vi "niRFSTS Sequence Flow Obtain Session.vi"(0 "Session  Name ()":string, 1 "Include All Evaluations?":bool, 2 "Prepend Result Names?":bool, 5 "New Sequence File Path":path=path "C:/Users/QFE3320 VM/Desktop/CW1.seq", 7 "Template Path":path=path "C:/QFE3320/QFE3320_Template.seq", 9 "Limits File Path":path, 11 "error in (no error)":errorcluster, 12 "Use Existing Test Numbers?":bool) -> (4 "Session Handle":T1, 15 "error out":errorcluster)   [LabVIEW 2018, in "niRFSTS Sequence Flow.lvclass"]
doc: "This function initializes the measurement\n\nPass the function a name to obtain an active measurement handle"
uses:
  niRFSTS Sequence Flow.lvclass
  Typedefs/Session Handle.ctl
  C:/Sequence Automation/Plugins/Sequence Automation Session.lvlibp/Sequence Automation Session.lvclass
  niRFSTS Sequence Flow.lvclass/niRFSTS Sequence Flow.ctl
  Plugins/Sequence Automation Session.lvlibp/Sequence Automation Session.lvclass
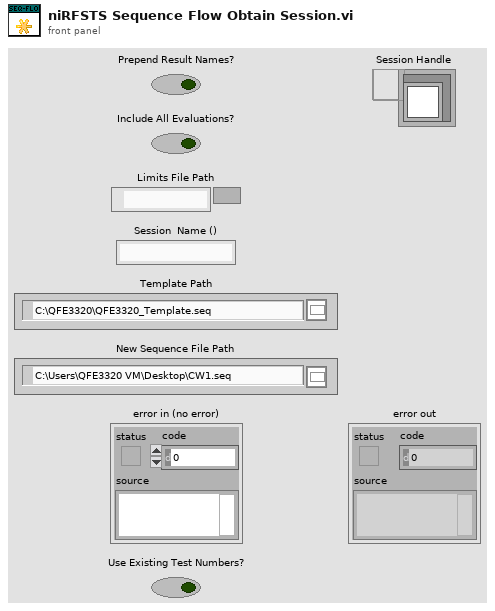
[diagram p1: front panel]
types:
  T1 = typedef "niRFSTS Sequence Flow.lvclass/Session Handle.ctl" = refnum<data-value>
  T2 = typedef "Sequence Automation Session.lvlibp/Sequence Automation Session.lvclass/Session Handle.ctl" = refnum<data-value>
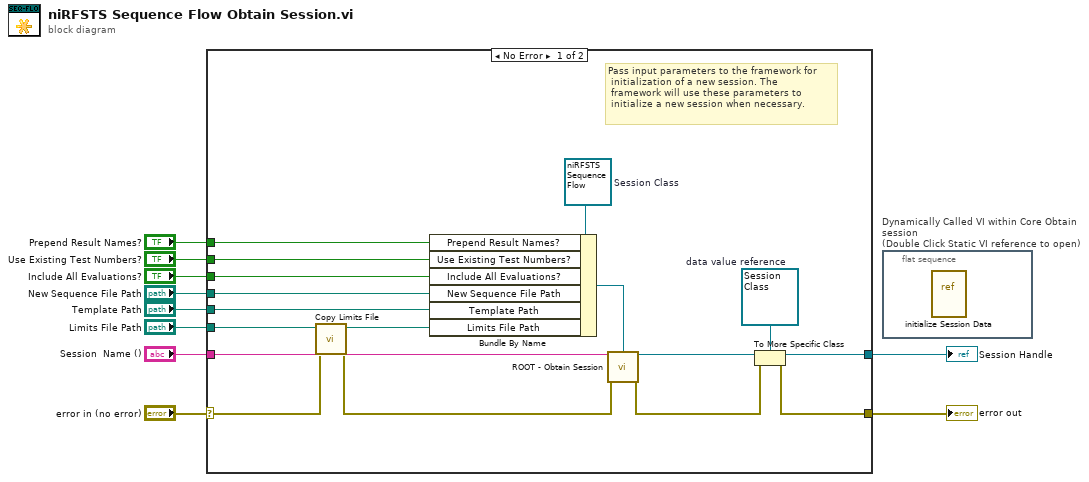
[diagram p0: block diagram]
diagram:
  n1 = case shown="No Error" "error in (no error)" {
    selector: "error in (no error)" -> [w11 w28]
    tunnel: [w25 w28] -> w9
    tunnel: [w26 _] -> w7
    tunnel: "Session  Name ()" -> [w27 _]
    tunnel: "New Sequence File Path" -> [w24 _]
    tunnel: "Template Path" -> [w23 _]
    tunnel: "Limits File Path" -> [w13 _]
    tunnel: "Use Existing Test Numbers?" -> [w22 _]
    tunnel: "Include All Evaluations?" -> [w19 _]
    tunnel: "Prepend Result Names?" -> [w21 _]
    frame No Error {
      w16 = refnum<data-value> refnum  # data value reference
      w15 = refnum<class "niRFSTS Sequence Flow.lvclass"> refnum  # Session Class
      # "Pass input parameters to the framework for\n initialization of a new session. The\n framework will use these parameters to\n initialize a new session when necessary."
      n2 = call "Copy Limits File.vi"("error in (no error)"=w11, "Limits File Path In"=w13) -> ("error out"=w20:errorcluster, "Limits File Path Out"=w12:path)  [unwired: 8 in]
      n3 = Bundle By Name(cluster=w15, "Prepend Result Names?"=w21, "Use Existing Test Numbers?"=w22, "Include All Evaluations?"=w19, "New Sequence File Path"=w24, "Template Path"=w23, "Limits File Path"=w12) -> (w14:refnum<class "niRFSTS Sequence Flow.lvclass">)
      n4 = call "ROOT - Obtain Session.vi"("Session Name ()"=w27, "OBJ - Session"=w14, "error in (no error)"=w20) -> ("Session Handle"=w17:T2, "error out"=w18:errorcluster)  [unwired: 10 in, 1 out]
      n5 = To More Specific Class(target class=w16, reference=w17, error in=w18) -> (specific class reference=w26:refnum<data-value>, error out=w25:errorcluster)
    }
    frame Error {
    }
  }
  "error out" <- w9
  "Session Handle" <- w7
  n6 = flat-sequence "Dynamically Called VI within Core Obtain session\n(Double Click Static VI reference to open)" {
    frame #0 {
      n7 = vi-ref "initialize Session Data.vi"() -> ()  [unwired: 1 out]
    }
  }
